vi "Create Element Output Power Supply.vi"(0 "Current Max SP":dbl, 1 "Current In":dbl, 2 "Current Min SP":dbl, 3 "Voltage Max SP":dbl, 4 "Voltage In":dbl, 5 "Voltage Min SP":dbl, 6 "Power Max SP":dbl, 7 "Power In":dbl, 8 "Error ACT":bool, 9 "Power Min SP":dbl, 10 "OnOff ACT":bool, 11 "Output Enable ACT":bool, 13 "Feedback In":bool) -> (20 "Current Out":dbl, 21 "Voltage Out":dbl, 22 "Power Out":dbl, 23 "Error Channels":i32, 24 "Feedback Out":bool)   [LabVIEW 2023]
uses:
  <vilib>/numeric/Random Number (Range) DBL.vi
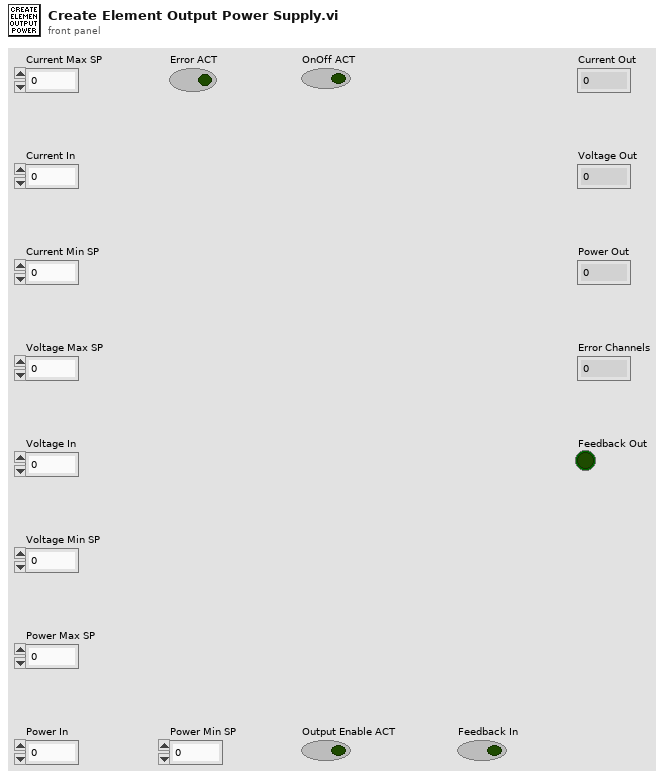
[diagram p1: front panel]
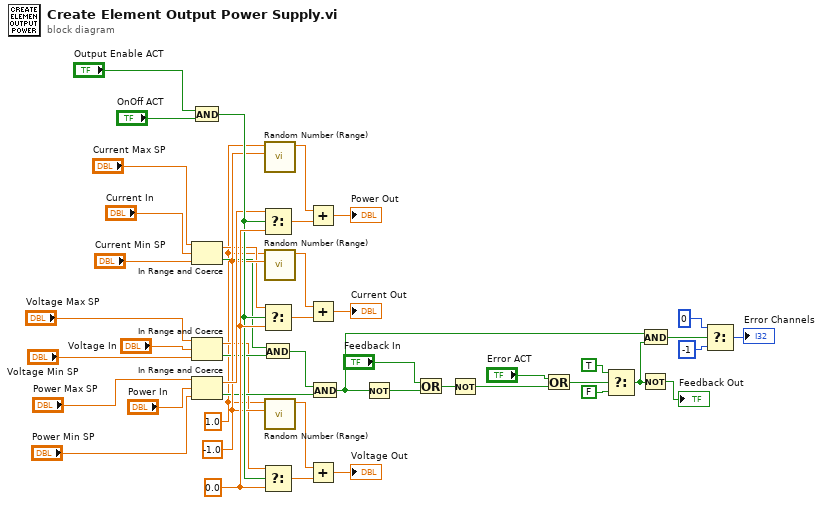
[diagram p0: block diagram]
diagram:
  w8 = 1.0 ("upper bound (100)")
  w21 = -1.0 ("lower bound (0)")
  w30 = 0.0 ("f")
  n1 = And(x="Output Enable ACT", y="OnOff ACT") -> (x .and. y?=w29:bool)
  n2 = In Range and Coerce(upper limit="Current Max SP", x="Current In", lower limit="Current Min SP") -> (coerced(x)=w13:dbl, In Range?=w19:bool)
  n3 = In Range and Coerce(upper limit="Voltage Max SP", x="Voltage In", lower limit="Voltage Min SP") -> (coerced(x)=w9:dbl, In Range?=w20:bool)
  n4 = In Range and Coerce(upper limit="Power Max SP", x="Power In", lower limit="Power Min SP") -> (coerced(x)=w28:dbl, In Range?=w18:bool)
  n5 = Select(t=w28, s=w29, f=w30) -> (s? t:f=w22:dbl)
  n6 = Select(t=w13, s=w29, f=w30) -> (s? t:f=w26:dbl)
  n7 = And(x=w19, y=w20) -> (x .and. y?=w17:bool)
  n8 = Select(t=w9, s=w29, f=w30) -> (s? t:f=w24:dbl)
  n9 = call-poly <vilib>:"Random Number (Range).vi"("lower bound (0)"=w21, "upper bound (100)"=w8) -> ("number"=w23:dbl)  [unwired: 9 in]
  n10 = call-poly <vilib>:"Random Number (Range).vi"("lower bound (0)"=w21, "upper bound (100)"=w8) -> ("number"=w27:dbl)  [unwired: 9 in]
  n11 = call-poly <vilib>:"Random Number (Range).vi"("lower bound (0)"=w21, "upper bound (100)"=w8) -> ("number"=w25:dbl)  [unwired: 9 in]
  n12 = Add(x=w23, y=w22) -> (x+y=→"Power Out":dbl)
  n13 = Add(x=w27, y=w26) -> (x+y=→"Current Out":dbl)
  n14 = Add(x=w25, y=w24) -> (x+y=→"Voltage Out":dbl)
  n15 = And(x=w17, y=w18) -> (x .and. y?=w6:bool)
  n16 = Not(x=w6) -> (.not. x?=w5:bool)
  n17 = Or(x="Feedback In", y=w5) -> (x .or. y?=w4:bool)
  n18 = Not(x=w4) -> (.not. x?=w3:bool)
  n19 = Or(x="Error ACT", y=w3) -> (x .or. y?=w12:bool)
  n20 = Select(t=TRUE, s=w12, f=FALSE) -> (s? t:f=w2:bool)
  n21 = Not(x=w2) -> (.not. x?=→"Feedback Out":bool)
  n22 = And(x=w6, y=w2) -> (x .and. y?=w16:bool)
  n23 = Select(t=0, s=w16, f=-1) -> (s? t:f=→"Error Channels":i32)
